vi "New_S2C_FORNAX_Proc_SendViper.vi"(8 "Error In":errorcluster, 11 "Q-Ref":refnum<queue>) -> (0 "Error Out":errorcluster)   [LabVIEW 2015]
uses:
  S2C_FORNAX_Proc_Globals.vi
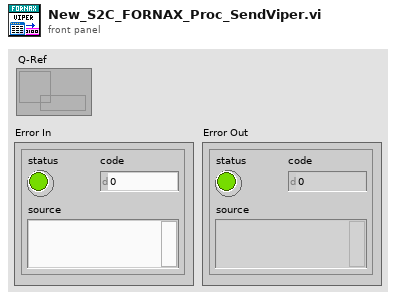
[diagram p1: front panel]
types:
  T1 = cluster{"Caller-Q":refnum<queue>, "Command":string, "Return":string, "Data":variant, "Timeout":dbl}
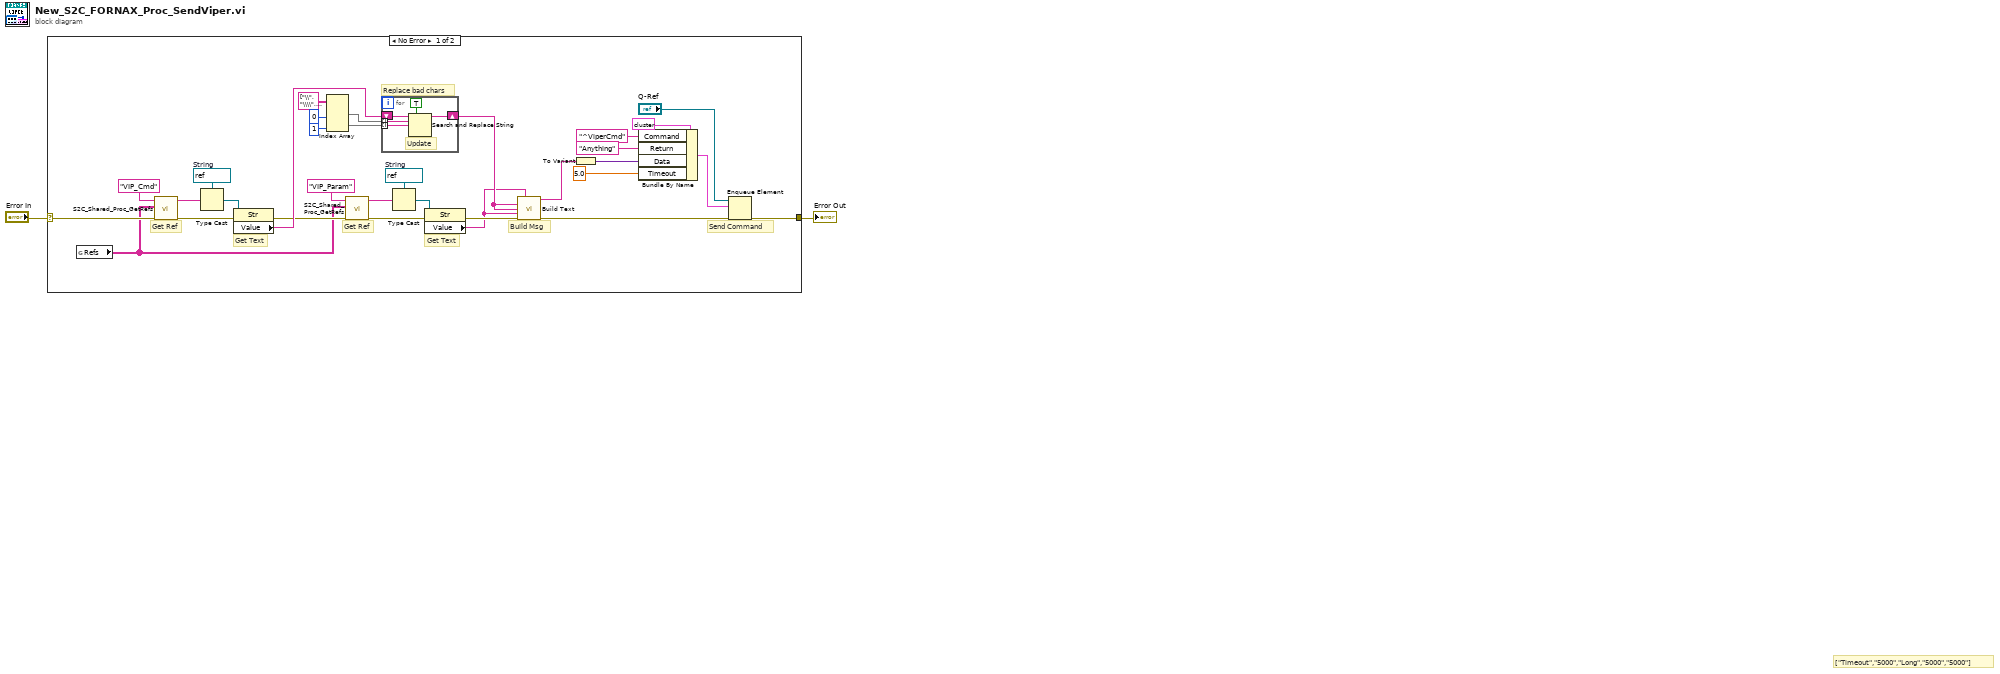
[diagram p0: block diagram]
diagram:
  # "[\"Timeout\",\"5000\",\"Long\",\"5000\",\"5000\"]"
  n1 = case shown="No Error" "Error In" {
    selector: "Error In" -> [w22 w40]
    tunnel: [w32 w40] -> w1
    frame No Error {
      w8 = refnum<vi> refnum  # String
      w29 = refnum<vi> refnum  # String
      # "Get Text"
      # "Get Ref"
      # "Get Text"
      # "Replace bad chars"
      # "Build Msg"
      # "Get Ref"
      # "Send Command"
      n2 = global read "S2C_FORNAX_Proc_Globals.vi" "Refs"() -> (w5:string[][])
      n3 = call "S2C_Shared_Proc_GetRefs.vi"("Error In"=w22, "Refs"=w5, "Label"="VIP_Cmd") -> ("Error Out"=w30:errorcluster, "Reference"=w28:string)  [unwired: 7 in]
      n4 = Type Cast(type=w29, x=w28) -> (*(type *) &x=w27:refnum<vi>)
      n5 = property class="Str"(reference=w27, error in=w30) -> (error out=w6:errorcluster, "Value"=w13:string)  [unwired: 1 out]
      n6 = Index Array(array=string[][] [["\\", "\\\\"], ["\"", "\\\""], ["\n", "\\n"], ["\r", "\\r"], ["\t", "\\t"]], index (col) #1=0 ("disabled index (col)"), index (col) #2=1 ("index (col)")) -> (element #1=w19:string[], element #2=w20:string[])  [unwired: 2 in]
      n7 = call "S2C_Shared_Proc_GetRefs.vi"("Error In"=w6, "Refs"=w5, "Label"="VIP_Param") -> ("Error Out"=w7:errorcluster, "Reference"=w9:string)  [unwired: 7 in]
      n8 = for {
        tunnel: w19 -> [w38] mode=indexing
        tunnel: w20 -> [w36] mode=indexing
        shift-right: [w35] -> w12
        shift-left: w13 -> [w39]
        # "Update"
        n9 = Search and Replace String(replace all?=TRUE ("replace all? (F)"), input string=w39, search string=w38, replace string=w36) -> (result string=w35:string)  [unwired: 4 in, 3 out]
      }
      n10 = Type Cast(type=w8, x=w9) -> (*(type *) &x=w10:refnum<vi>)
      n11 = property class="Str"(reference=w10, error in=w7) -> (error out=w4:errorcluster, "Value"=w3:string)  [unwired: 1 out]
      n12 = call "Build Text"("Param1"=w3, "Cmd"=w12, "Cmd1"=w12, "Param"=w3, "error in (no error)"=w4) -> ("Result"=w15:string, "error out"=w14:errorcluster)  [unwired: 9 in]
      n13 = To Variant(anything=w15) -> (Variant=w25:variant)
      n14 = Bundle By Name(cluster=T1 {"Caller-Q"=refnum, "Command"="", "Return"="None", "Data"=variant, "Timeout"=10.0} ("element"), "Command"="^ViperCmd" ("string"), "Return"="Anything", "Data"=w25, "Timeout"=5.0) -> (w31:T1)
      n15 = Enqueue Element(queue="Q-Ref", element=w31, error in (no error)=w14) -> (error out=w32:errorcluster)  [unwired: 1 in, 2 out]
    }
    frame Error {
    }
  }
  "Error Out" <- w1
